vi "Get_Voices.vi"(4 "error out":errorcluster, 5 "OptionalAttributes":string, 6 "RequiredAttributes":string, 7 "SpeechLib.ISpeechVoice (In)":refnum<k7>) -> (0 "error out":errorcluster, 1 "Voice Names":string[](array[string]), 2 "GetVoices (Out)":refnum<k7>, 3 "SpeechLib.ISpeechVoice (Out)":refnum<k7>)   [LabVIEW 8.6]
doc: "This SubVI calls the Microsoft Speech SDK 5.1 software and loads the voices available into an output array for use by the LVTTS.vi"
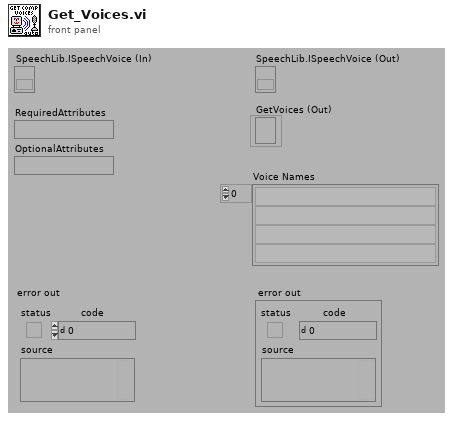
[diagram p1: front panel]
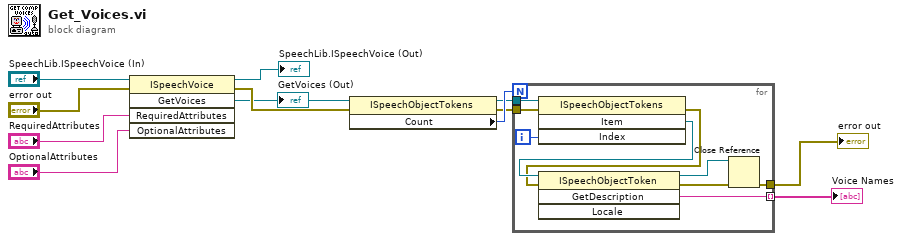
[diagram p0: block diagram]
diagram:
  n1 = invoke class="ISpeechVoice" method="GetVoices"(reference="SpeechLib.ISpeechVoice (In)", error in="error out", "RequiredAttributes"="RequiredAttributes", "OptionalAttributes"="OptionalAttributes") -> (reference out=→"SpeechLib.ISpeechVoice (Out)":refnum<k7>, error out=w7:errorcluster, "GetVoices"=w6:refnum<k7>)  [unwired: 1 in, 2 out]
  "GetVoices (Out)" <- w6
  n2 = property class="ISpeechObjectTokens"(reference=w6, error in=w7) -> (reference out=w9:refnum<k7>, error out=w8:errorcluster, "Count"=w10:i32)
  n3 = for {
    N: w10 -> [_]
    tunnel: [w13] -> w5
    tunnel: w8 -> [w18]
    tunnel: w9 -> [w17]
    tunnel: [w16] -> w11 mode=indexing
    i -> [w20]
    n4 = invoke class="ISpeechObjectTokens" method="Item"(reference=w17, error in=w18, "Index"=w20) -> (error out=w15:errorcluster, "Item"=w21:refnum<k7>)  [unwired: 1 in, 2 out]
    n5 = invoke class="ISpeechObjectToken" method="GetDescription"(reference=w21, error in=w15) -> (reference out=w19:refnum<k7>, error out=w14:errorcluster, "GetDescription"=w16:string)  [unwired: 2 in, 1 out]
    n6 = Close Reference(reference=w19, error in (no error)=w14) -> (error out=w13:errorcluster)
  }
  "Voice Names" <- w11
  "error out" <- w5
